vi "vetorTeste.vi"() -> ()   [LabVIEW 2014]
panel:
  out "x+1":i32
  in  "stop":bool
  out "output array":dbl[](array[numeric])
  out "teste":dbl[](array[numeric])
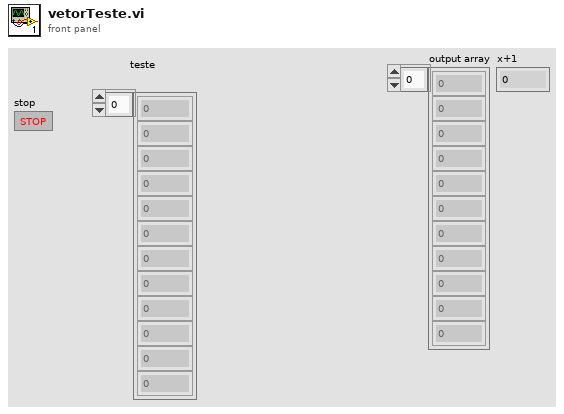
[diagram p1: front panel]
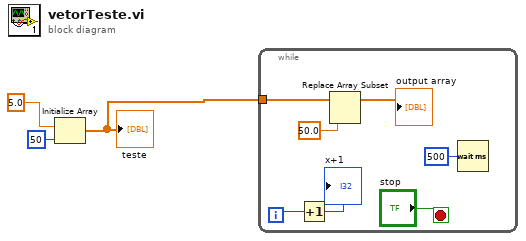
[diagram p0: block diagram]
diagram:
  n1 = Initialize Array(5.0 ("element"), 50 ("dimension size")) -> (w1:dbl[])
  "teste" <- w1
  n2 = while {
    tunnel: w1 -> [w6]
    i -> [w10]
    stop <- "stop" stop-if-true
    n3 = Increment(x=w10) -> (x+1=→"x+1":i32)
    n4 = Replace Array Subset(array=w6, new element=50.0 ("new element/subarray")) -> (→"output array":dbl[])  [unwired: 1 in]
    n5 = Wait (ms)(milliseconds to wait=u32 500) -> ()  [unwired: 1 out]
  }
